vi "fgv-data - log.vi"(7 "cmd":T1, 8 "error in":errorcluster, 11 "element":variant) -> (0 "error out":errorcluster, 3 "queue out":refnum<queue>)   [LabVIEW 2019]
uses:
  _ctrl/create-rw-close.ctl
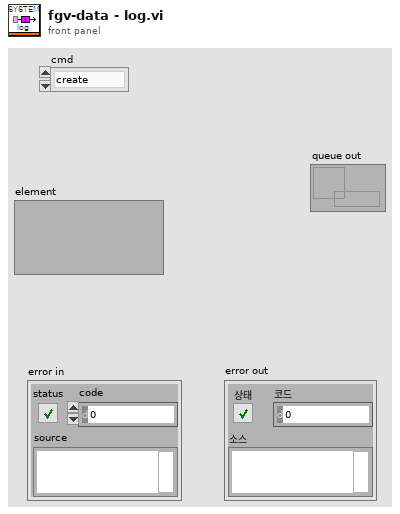
[diagram p1: front panel]
types:
  T1 = typedef "create-rw-close.ctl" = enum16{"create", "write", "read", "delete", "close"}
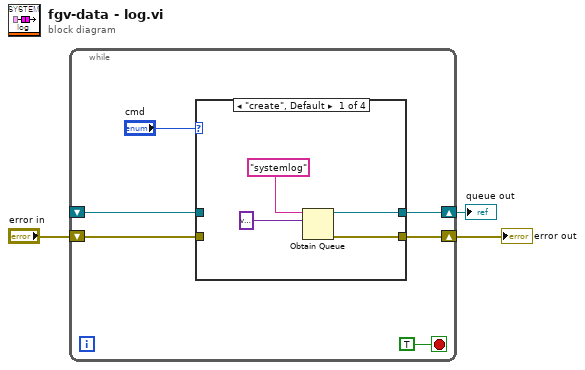
[diagram p0: block diagram]
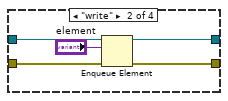
[diagram p2: hidden frame]
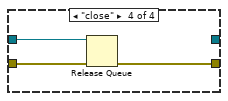
[diagram p4: hidden frame]
diagram:
  n1 = while {
    shift-right: [w7] -> w1
    shift-left: _ -> [w4]
    shift-right: [w6] -> w3
    shift-left: "error in" -> [w5]
    stop <- TRUE stop-if-true
    n2 = case shown="\"create\", Default" "cmd" {
      tunnel: [w13 w16 w20 _] -> w7
      tunnel: [w12 w17 w19 w22] -> w6
      tunnel: w5 -> [_ w18 w19 w23]
      tunnel: w4 -> [_ w15 w20 w21]
      frame "create", Default {
        n3 = Obtain Queue(name (unnamed)="systemlog" ("이름(이름없음)"), element data type=variant) -> (queue out=w13:refnum<queue>, error out=w12:errorcluster)  [unwired: 3 in, 1 out]
      }
      frame "write" {
        n4 = Enqueue Element(queue=w15, element="element", error in (no error)=w18) -> (queue out=w16:refnum<queue>, error out=w17:errorcluster)  [unwired: 1 in, 1 out]
      }
      frame "read" {
      }
      frame "close" {
        n5 = Release Queue(queue=w21, error in (no error)=w23) -> (error out=w22:errorcluster)  [unwired: 1 in, 2 out]
      }
    }
  }
  "error out" <- w3
  "queue out" <- w1
